vi "Read CtlRef.vi"(8 "error in (no error)":errorcluster, 11 "TreeEditCellMsg in":refnum<class "TreeEditCellMsg.lvclass">) -> (0 "error out":errorcluster, 2 "CtlRef":refnum<vi>, 3 "TreeEditCellMsg out":refnum<class "TreeEditCellMsg.lvclass">)   [LabVIEW 2019, in "ActorEvents.lvlib" / "TreeEditCellMsg.lvclass"]
uses:
  <vilib>/gpm_packages/@cs/mva-viewable/Source/ActorEvents/IEventAggregator Messages/TreeEditCellMsg/TreeEditCellMsg.lvclass
  <vilib>/gpm_packages/@cs/mva-viewable/Source/ActorEvents/IEventAggregator Messages/TreeEditCellMsg/TreeEditCellMsg.lvclass/TreeEditCellMsg.ctl
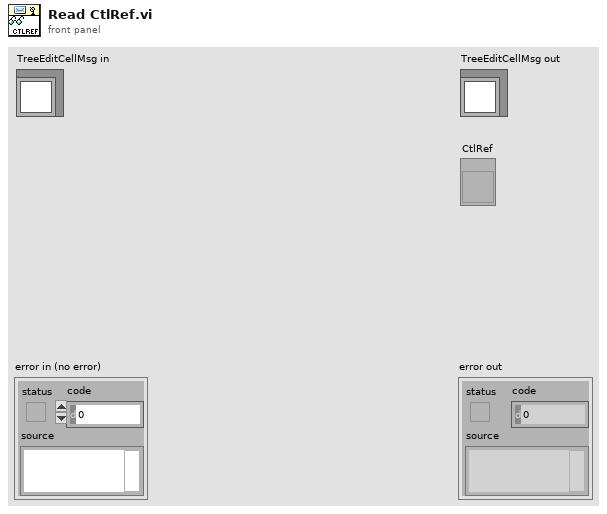
[diagram p1: front panel]
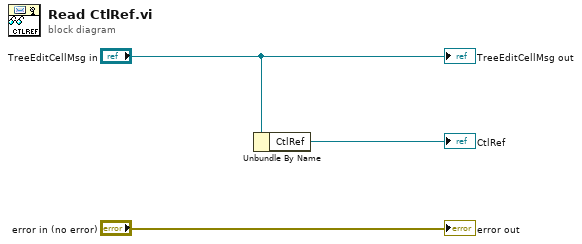
[diagram p0: block diagram]
diagram:
  n1 = Unbundle By Name("TreeEditCellMsg in") -> ("CtlRef"=→"CtlRef":refnum<vi>)
  "error out" <- "error in (no error)"
  "TreeEditCellMsg out" <- "TreeEditCellMsg in"
